vi "Ref_Num_Stopwatch_Op.vi"(0 "Elapsed time (seconds)":refnum<vi>, 2 "start time":refnum<vi>, 3 "Started":refnum<vi>, 4 "OK Button":refnum<vi>, 5 "stop":refnum<vi>) -> ()   [LabVIEW 2020]
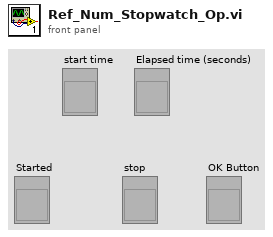
[diagram p1: front panel]
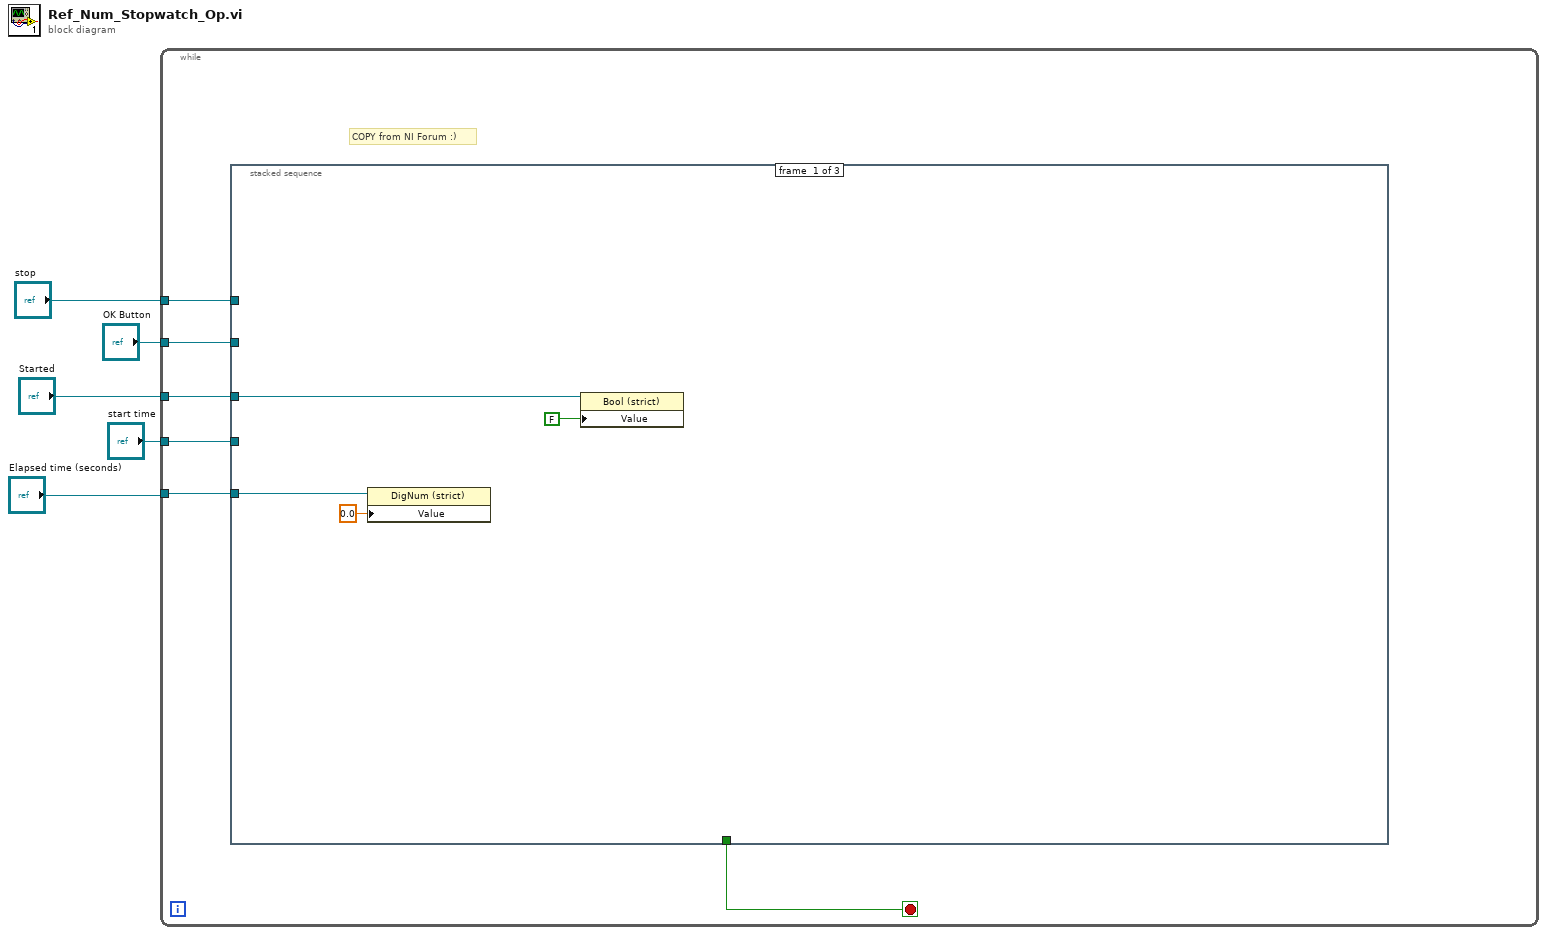
[diagram p0: block diagram]
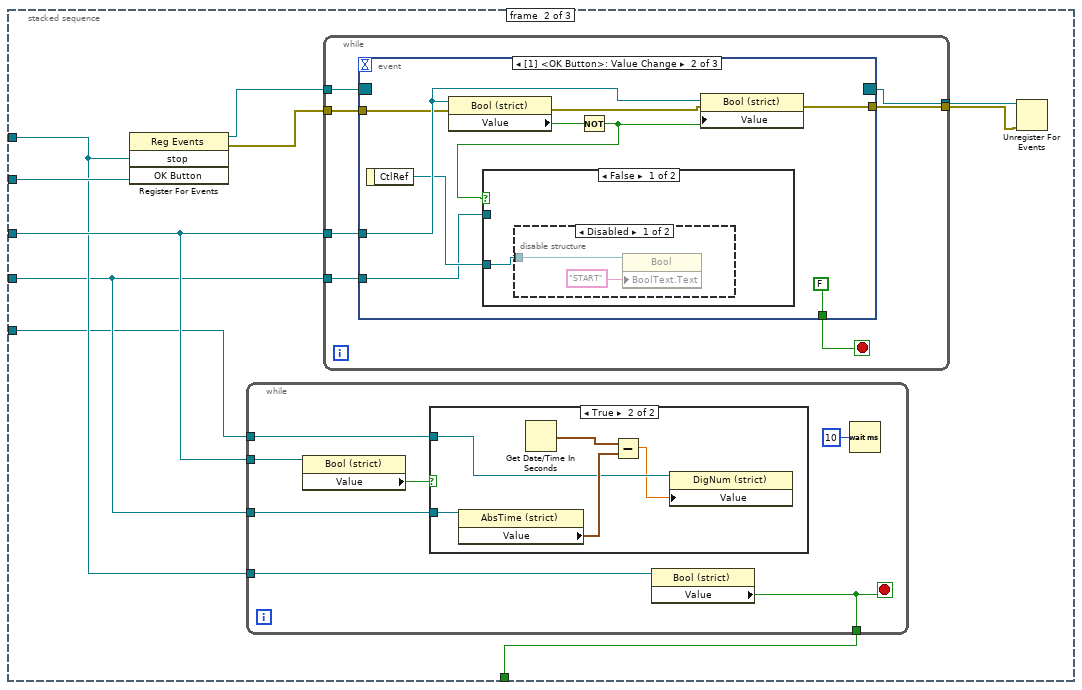
[diagram p2: hidden frame]
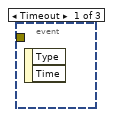
[diagram p4: hidden frame]
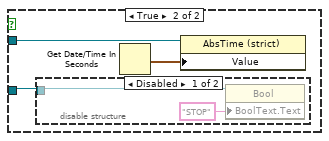
[diagram p6: hidden frame]
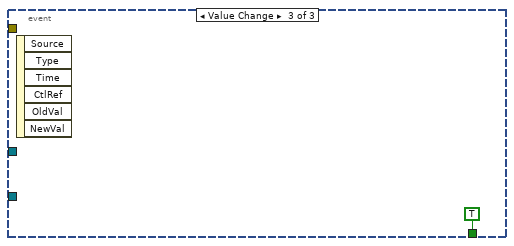
[diagram p8: hidden frame]
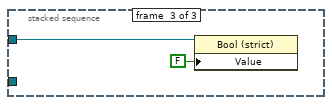
[diagram p9: hidden frame]
diagram:
  n1 = while {
    tunnel: "Started" -> [w11]
    tunnel: "OK Button" -> [w10]
    tunnel: "Elapsed time (seconds)" -> [w9]
    tunnel: "stop" -> [w8]
    tunnel: "start time" -> [w7]
    stop <- w6 stop-if-true
    # "COPY from NI Forum :)"
    n2 = stacked-sequence {
      tunnel: [_ w25 _] -> w6
      tunnel: w11 -> [w15 w22 _]
      tunnel: w10 -> [_ w24 _]
      tunnel: w9 -> [w13 w19 _]
      tunnel: w8 -> [_ w21 w64]
      tunnel: w7 -> [_ w20 _]
      frame #0 {
        n3 = property class="DigNum (strict)"(reference=w13, "Value"=0.0 ("Elapsed time (seconds)")) -> ()  [unwired: 1 in, 2 out]
        n4 = property class="Bool (strict)"(reference=w15, "Value"=FALSE ("Started")) -> ()  [unwired: 1 in, 2 out]
      }
      frame #1 {
        n5 = register-events(w21, w24) -> (reference out=w23:refnum<event-registration>, error out=w17:errorcluster)  [unwired: 2 in]
        n6 = while {
          tunnel: [w28] -> w25
          tunnel: w22 -> [w31]
          tunnel: w21 -> [w29]
          tunnel: w20 -> [w27]
          tunnel: w19 -> [w26]
          stop <- w28 stop-if-true
          n7 = property class="Bool (strict)"(reference=w31) -> ("Value"=w30:bool)  [unwired: 1 in, 2 out]
          n8 = case shown="True" w30 {
            tunnel: w27 -> [_ w36]
            tunnel: w26 -> [_ w34]
            frame False {
              # "do nothing"
            }
            frame True {
              n9 = property class="AbsTime (strict)"(reference=w36) -> ("Value"=w35:timestamp)  [unwired: 1 in, 2 out]
              n10 = Get Date/Time In Seconds() -> (seconds since 1Jan1904=w37:timestamp)
              n11 = Subtract(x=w37, y=w35) -> (x-y=w33:dbl)
              n12 = property class="DigNum (strict)"(reference=w34, "Value"=w33) -> ()  [unwired: 1 in, 2 out]
            }
          }
          n13 = property class="Bool (strict)"(reference=w29) -> ("Value"=w28:bool)  [unwired: 1 in, 2 out]
          n14 = Wait (ms)(milliseconds to wait=u32 10) -> ()  [unwired: 1 out]
        }
        n15 = while {
          tunnel: w23 -> [w43]
          tunnel: w22 -> [w42]
          tunnel: w20 -> [w41]
          tunnel: [w40] -> w18
          tunnel: w17 -> [w39]
          tunnel: [w38] -> w16
          stop <- w44 stop-if-true
          n16 = event shown="[1] <OK Button>: Value Change" {
            selector: w43 -> [_ _ _]
            dyn-events: [_ _ _] -> w40
            timeout: _ -> [_ _ _]
            tunnel: [_ FALSE TRUE] -> w44
            tunnel: w42 -> [_ w52 _]
            tunnel: w41 -> [_ w48 _]
            tunnel: w39 -> [_ w47 _]
            tunnel: [_ w45 _] -> w38
            event Timeout {
              n17 = event-data() -> ()  [unwired: 1 in, 2 out]
            }
            event Value Change {
              n18 = event-data() -> ("CtlRef"=w49:refnum<vi>)  [unwired: 1 in]
              n19 = property class="Bool (strict)"(reference=w52, error in=w47) -> (error out=w46:errorcluster, "Value"=w51:bool)  [unwired: 1 out]
              n20 = Not(x=w51) -> (.not. x?=w50:bool)
              n21 = case shown="False" w50 {
                tunnel: w49 -> [w54 w59]
                tunnel: w48 -> [_ w58]
                frame False {
                  n22 = disable-structure shown="Disabled" {
                    disable-tunnel: w54 -> [w56 _]
                    frame Disabled {
                      n23 = property class="Bool"(reference=w56, "BoolText.Text"="START" ("Caption.Text")) -> ()  [unwired: 1 in, 2 out]
                    }
                    frame Enabled {
                    }
                  }
                }
                frame True {
                  n24 = disable-structure shown="Disabled" {
                    disable-tunnel: w59 -> [w60 _]
                    frame Disabled {
                      n25 = property class="Bool"(reference=w60, "BoolText.Text"="STOP" ("Caption.Text")) -> ()  [unwired: 1 in, 2 out]
                    }
                    frame Enabled {
                    }
                  }
                  n26 = Get Date/Time In Seconds() -> (seconds since 1Jan1904=w57:timestamp)
                  n27 = property class="AbsTime (strict)"(reference=w58, "Value"=w57) -> ()  [unwired: 1 in, 2 out]
                }
              }
              n28 = property class="Bool (strict)"(reference=w52, error in=w46, "Value"=w50) -> (error out=w45:errorcluster)  [unwired: 1 out]
            }
            event Value Change {
              n29 = event-data() -> ()  [unwired: 1 in, 6 out]
            }
          }
        }
        n30 = Unregister For Events(event registration refnum=w18, error in=w16) -> ()  [unwired: 1 out]
      }
      frame #2 {
        n31 = property class="Bool (strict)"(reference=w64, "Value"=FALSE) -> ()  [unwired: 1 in, 2 out]
      }
    }
  }
